vi "utility.Hash.vi"(8 "错误输入（无错误）":errorcluster, 10 "Hash_Mode":enum16{"SHA1", "SHA256", "SHA384", "SHA512"}(ring), 11 "Input":string) -> (0 "错误输出":errorcluster, 2 "Length":i32, 3 "Hash_Code":string)   [LabVIEW 2012, in "Lib_UEL.ATE.lvlib" / "Lib_App.lvlib"]
uses:
  Lib_App.lvlib
  D:/MyWork/MyWork/Labview_Lib/App/hash.dll
  hash.dll
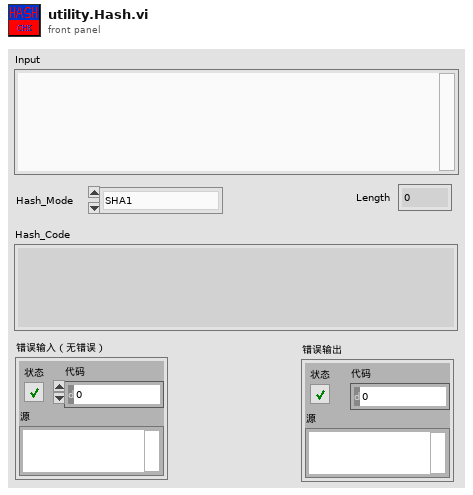
[diagram p1: front panel]
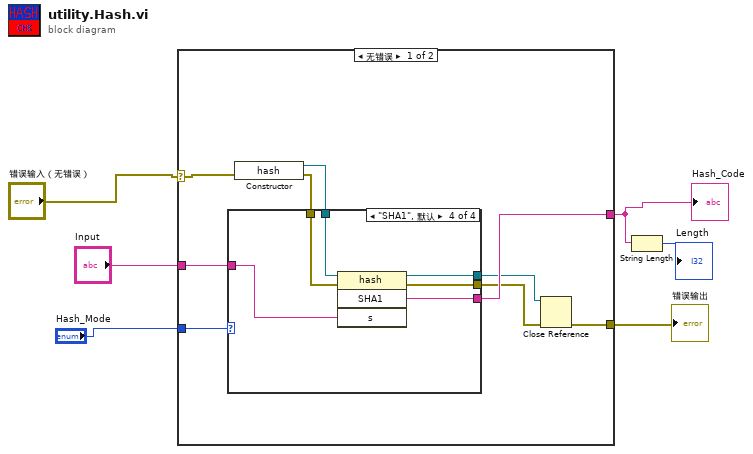
[diagram p0: block diagram]
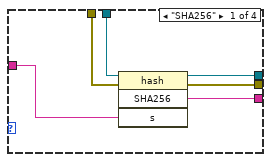
[diagram p2: hidden frame]
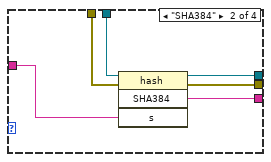
[diagram p3: hidden frame]
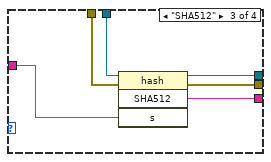
[diagram p4: hidden frame]
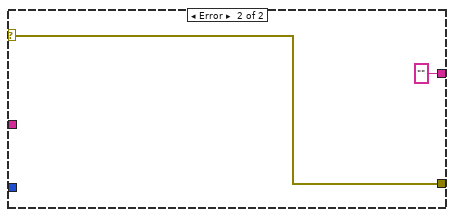
[diagram p5: hidden frame]
diagram:
  n1 = case shown="无错误" "错误输入（无错误）" {
    selector: "错误输入（无错误）" -> [w12 w40]
    tunnel: [w15 "" ("SHA256")] -> w6
    tunnel: "Input" -> [w14 _]
    tunnel: [w9 w40] -> w2
    tunnel: "Hash_Mode" -> [w8 _]
    frame No Error {
      n2 = constructor class="hash"(error in=w12) -> (reference out=w7:refnum<k24>, error out=w13:errorcluster)  [unwired: 2 in, 1 out]
      n3 = case shown="\"SHA1\", 默认" w8 {
        tunnel: w7 -> [w21 w27 w33 w39]
        tunnel: [w20 w26 w32 w38] -> w15
        tunnel: w14 -> [w19 w25 w31 w37]
        tunnel: w13 -> [w18 w24 w30 w36]
        tunnel: [w17 w23 w29 w35] -> w11
        tunnel: [w16 w22 w28 w34] -> w10
        frame "SHA256" {
          n4 = invoke on="调用节点" class="hash" method="SHA256"(reference=w21, error in=w18, "s"=w19) -> (reference out=w17:refnum<k24>, error out=w16:errorcluster, "SHA256"=w20:string)  [unwired: 1 in, 1 out]
        }
        frame "SHA384" {
          n5 = invoke on="调用节点" class="hash" method="SHA384"(reference=w27, error in=w24, "s"=w25) -> (reference out=w23:refnum<k24>, error out=w22:errorcluster, "SHA384"=w26:string)  [unwired: 1 in, 1 out]
        }
        frame "SHA512" {
          n6 = invoke on="调用节点" class="hash" method="SHA512"(reference=w33, error in=w30, "s"=w31) -> (reference out=w29:refnum<k24>, error out=w28:errorcluster, "SHA512"=w32:string)  [unwired: 1 in, 1 out]
        }
        frame "SHA1", Default {
          n7 = invoke on="调用节点" class="hash" method="SHA1"(reference=w39, error in=w36, "s"=w37) -> (reference out=w35:refnum<k24>, error out=w34:errorcluster, "SHA1"=w38:string)  [unwired: 1 in, 1 out]
        }
      }
      n8 = Close Reference(reference=w11, error in (no error)=w10) -> (error out=w9:errorcluster)
    }
    frame Error {
    }
  }
  "Hash_Code" <- w6
  "错误输出" <- w2
  n9 = String Length(string=w6) -> (length=→"Length":i32)
